vi "Wire Controls to Mock Call.vi"(8 "error in (no error)":errorcluster, 10 "Controls":map{string, refnum<vi>}(c390), 11 "VI in":refnum<vi>) -> (0 "error out":errorcluster, 3 "VI out":refnum<vi>)   [LabVIEW 2020, in "Pure Mock Class Generator.lvclass"]
uses:
  Pure Mock Class Generator.lvclass
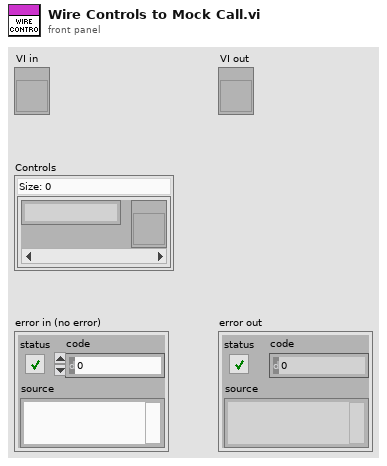
[diagram p1: front panel]
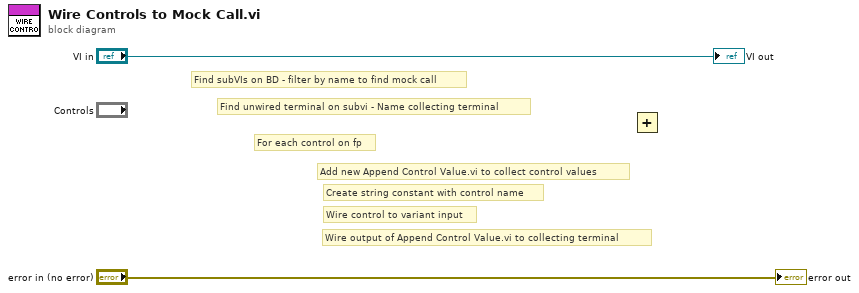
[diagram p0: block diagram]
diagram:
  # "Wire control to variant input"
  # "Create string constant with control name"
  # "Wire output of Append Control Value.vi to collecting terminal"
  # "For each control on fp"
  # "Add new Append Control Value.vi to collect control values"
  # "Find unwired terminal on subvi - Name collecting terminal"
  # "Find subVIs on BD - filter by name to find mock call"
  n1 = Add() -> ()  [unwired: 2 in, 1 out]
  "error out" <- "error in (no error)"
  "VI out" <- "VI in"
